vi "Michael_DisplaySLM.vi"(10 "weight SLMB":dbl=1.0, 11 "weight SLM A":dbl=1.0) -> ()   [LabVIEW 2015]
uses:
  <userlib>/TAM_Program/TAM Sub VIs.llb/BaseHologramGlobal.vi
panel:
  out "Intensity Graph":dbl[][](graph)
  in  "stop":bool
  out "max value":dbl=0.0002545111260339989
  in  "Load global\nbase parameters?":bool=TRUE
  in  "Base hologram parameters":T1={"x centre A (m)"=0.00023877834010536838, "y centre A (m)"=-1.0895093102686923e-05, "x angle A (mrad)"=10.0, "y angle A (mrad)"=0.0, "f lens A (m)"=1000000.0, "x centre B (m)"=-0.00031192399117047087, "y centre B (m)"=-0.00028507383868835634, "x angle B (mrad)"=10.0, "y angle B (mrad)"=0.0, "f lens B (m)"=1000000.0} {"f lens B (m)" format="%_3g"; "y angle B (mrad)" format="%_8g"; "x angle B (mrad)" format="%_8g"; "y centre B (m)" format="%_8p"; "x centre B (m)" format="%_8p"; "f lens A (m)" format="%_3g"; "y angle A (mrad)" format="%_8g"; "x angle A (mrad)" format="%_8g"; "y centre A (m)" format="%_8p"; "x centre A (m)" format="%_8p"}
  in  "beam waist w0 (m)":dbl=0.0005 format="%_3p"
  out "Hologram A":u8[][](graph)
  out "Hologram B":u8[][](graph)
  in  "mode B":T2(array[cluster])=[{"type"=enum."LG mode", "m or L"=0, "n or p"=0, "weight"=1.0, "phase"=0.0}]
  in  "mode A":T2(array[cluster])=[{"type"=enum."LG mode", "m or L"=0, "n or p"=0, "weight"=1.0, "phase"=0.0}]
  # "Set global\nbase parameters?"
  # "to account for \nunequal efficiencies,\nset to 1 if not intensity masking"
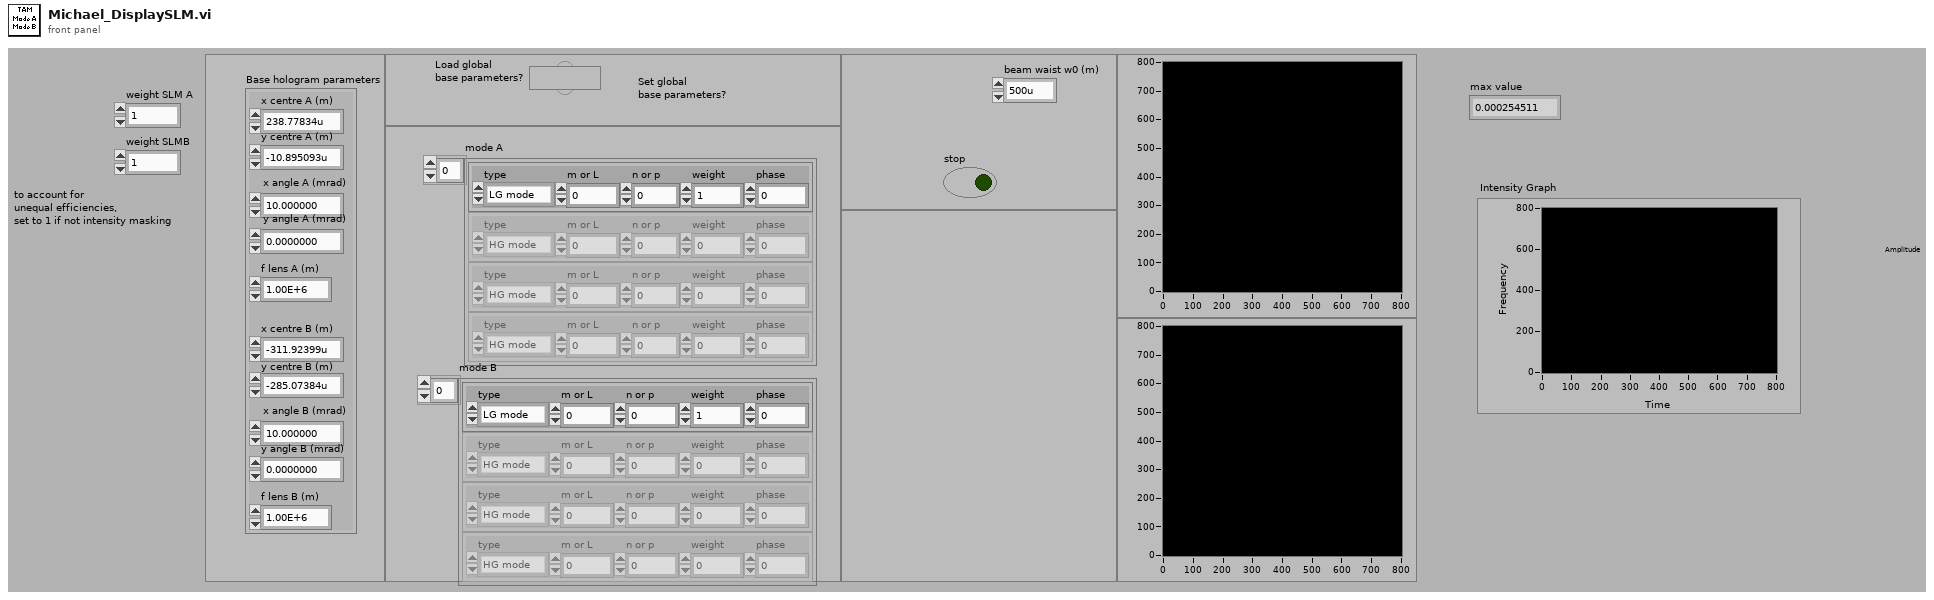
[diagram p1: front panel]
types:
  T1 = cluster{"x centre A (m)":dbl, "y centre A (m)":dbl, "x angle A (mrad)":dbl, "y angle A (mrad)":dbl, "f lens A (m)":dbl, "x centre B (m)":dbl, "y centre B (m)":dbl, "x angle B (mrad)":dbl, "y angle B (mrad)":dbl, "f lens B (m)":dbl}
  T2 = cluster{"type":enum16{"HG mode", "LG mode"}, "m or L":i32, "n or p":i32, "weight":dbl, "phase":dbl}[]
  T3 = cluster{"amplitude matrix":cdb[][], "number of columns in amplitude matrix":i32, "number of rows in amplitude matrix":i32, "represented width (in m)":dbl, "represented height (in m)":dbl, "wavelength (in m)":dbl}
  T4 = cluster{"type":enum16{"HG mode", "LG mode"}, "m or L":i32, "n or p":i32, "weight":dbl, "phase":dbl}
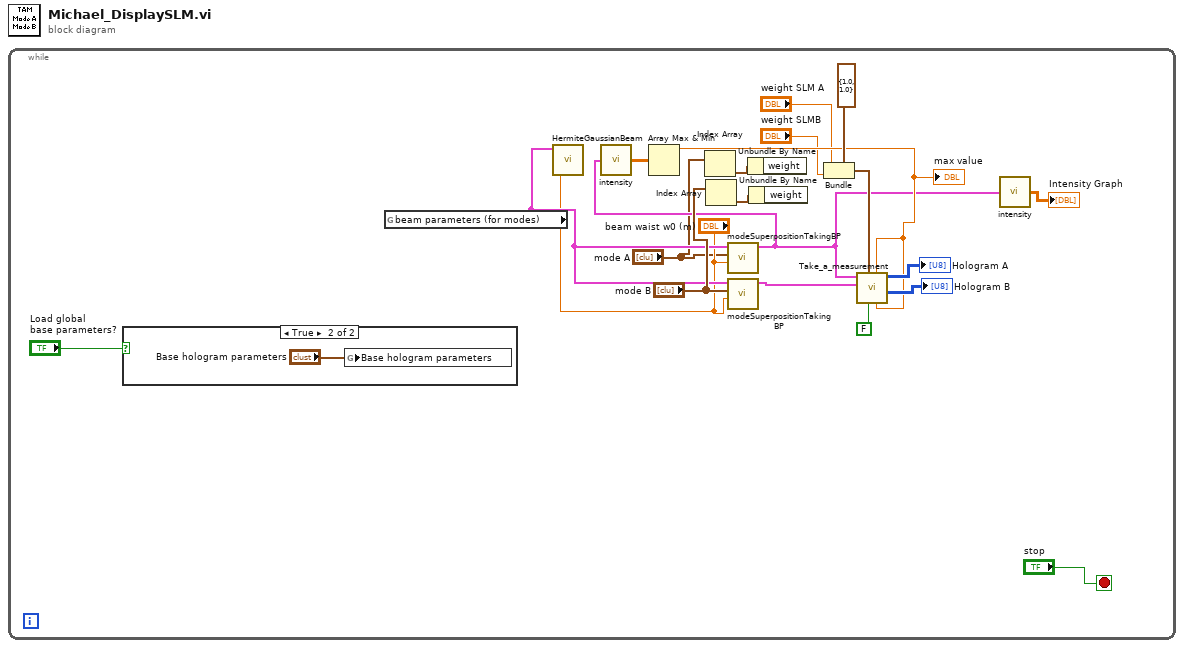
[diagram p0: block diagram]
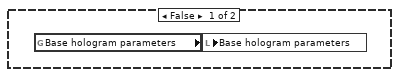
[diagram p2: hidden frame]
diagram:
  n1 = while {
    stop <- "stop" stop-if-true
    n2 = case shown="True" "Load global\nbase parameters?" {
      frame False {
        n3 = global read "BaseHologramGlobal.vi" "Base hologram parameters"() -> (w21:T1)
        n4 = local write "Base hologram parameters"(w21) -> ()
      }
      frame True {
        n5 = global write "BaseHologramGlobal.vi" "Base hologram parameters"("Base hologram parameters") -> ()
      }
    }
    n6 = global read "BaseHologramGlobal.vi" "beam parameters (for modes)"() -> (w11:T3)
    n7 = call <userlib>:"HermiteGaussianBeam.vi"("beam waist w0 (in m; default 1E-4 = 0.1mm)"="beam waist w0 (m)", "beam parameters"=w11) -> ()  [unwired: 4 in, 1 out]
    n8 = Index Array(array="mode A") -> (element=w15:T4)  [unwired: 1 in]
    n9 = Index Array(array="mode B") -> (element=w14:T4)  [unwired: 1 in]
    n10 = call <userlib>:"modeSuperpositionTakingBP.vi"("beam waist w0 (in m; default 1E-4 = 0.1mm)"="beam waist w0 (m)", "modes"="mode A", "beam parameters"=w11) -> ("mode superposition"=w3:T3)  [unwired: 8 in]
    n11 = call <userlib>:"intensity.vi"("beam cluster"=w3) -> ("intensity matrix"=w9:dbl[][])
    n12 = Array Max & Min(array=w9) -> (max value=w7:dbl)  [unwired: 3 out]
    "max value" <- w7
    n13 = call <userlib>:"modeSuperpositionTakingBP.vi"("beam waist w0 (in m; default 1E-4 = 0.1mm)"="beam waist w0 (m)", "modes"="mode B", "beam parameters"=w11) -> ("mode superposition"=w12:T3)  [unwired: 8 in]
    n14 = Unbundle By Name(w15) -> ()  [unwired: 1 out]
    n15 = Unbundle By Name(w14) -> ()  [unwired: 1 out]
    n16 = Bundle(cluster=cluster{"weight A":dbl, "weight B":dbl} {"weight A"=1.0, "weight B"=1.0} ("Weights for SLM"), "weight A"="weight SLM A", "weight B"="weight SLMB") -> (w16:cluster{"weight A":dbl, "weight B":dbl})
    n17 = call <userlib>:"Take_a_measurement.vi"("ref intensity B"=w7, "ref intensity A"=w7, "Use ref. intensity"=FALSE, "Weights for SLM"=w16, "Mode B"=w12, "Mode A"=w3) -> ("Hologram B"=→"Hologram B":u8[][], "Hologram A"=→"Hologram A":u8[][])  [unwired: 4 in]
    n18 = call <userlib>:"intensity.vi"("beam cluster"=w3) -> ("intensity matrix"=→"Intensity Graph":dbl[][])
  }
